vi "Ramp up.vi"(7 "ramp up speed":dbl, 8 "shift in":dbl, 9 "min":dbl, 10 "max":dbl, 11 "Ramp up/down":bool) -> (0 "shift out / output":dbl)   [LabVIEW 2014]
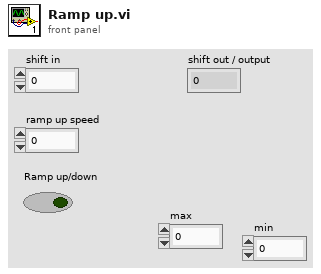
[diagram p1: front panel]
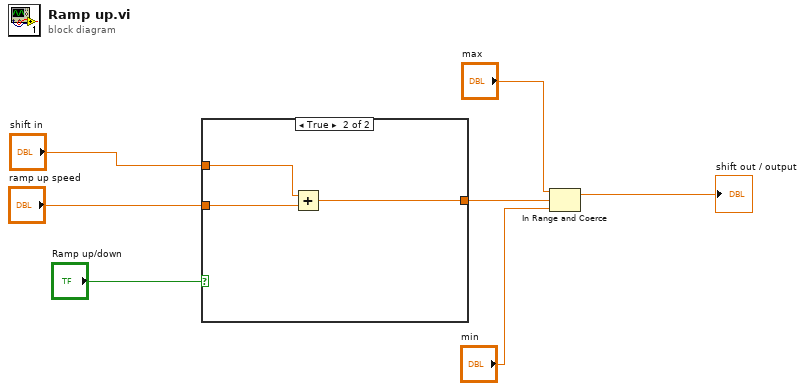
[diagram p0: block diagram]
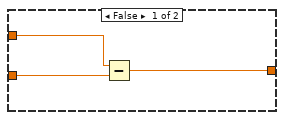
[diagram p2: hidden frame]
diagram:
  n1 = case shown="True" "Ramp up/down" {
    tunnel: "shift in" -> [w10 w13]
    tunnel: "ramp up speed" -> [w9 w12]
    tunnel: [w8 w11] -> w4
    frame False {
      n2 = Subtract(x=w10, y=w9) -> (x-y=w8:dbl)
    }
    frame True {
      n3 = Add(x=w13, y=w12) -> (x+y=w11:dbl)
    }
  }
  n4 = In Range and Coerce(upper limit="max", x=w4, lower limit="min") -> (coerced(x)=→"shift out / output":dbl)  [unwired: 1 out]
